vi "Write_Spreadsheet.vi"(0 "File_Path":path, 7 "Table":string[][](array[string]), 11 "Error_In":errorcluster) -> (15 "Error_Out":errorcluster)   [LabVIEW 2023, in "Custom_Sort_Library.lvlib"]
doc: "This VI Writes the given data to CSV file"
uses:
  Custom_Sort_Library.lvlib
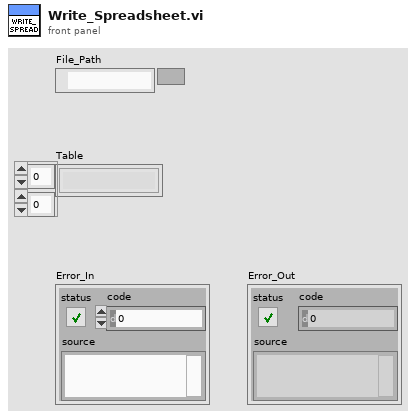
[diagram p1: front panel]
types:
  T1 = enum16{"open", "replace", "create", "open or create", "replace or create", "replace or create with confirmation"}
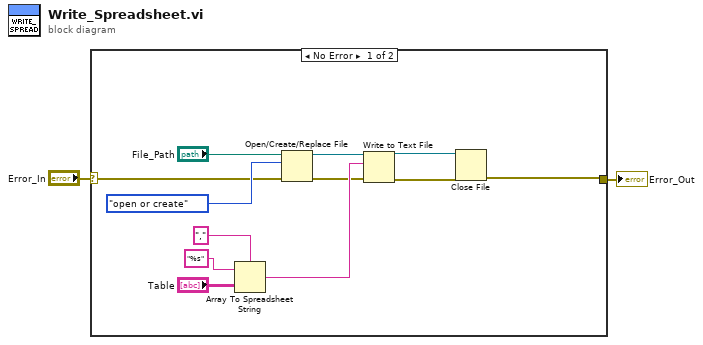
[diagram p0: block diagram]
diagram:
  n1 = case shown="No Error" "Error_In" {
    selector: "Error_In" -> [w9 w15]
    tunnel: [w4 w15] -> w2
    frame No Error {
      n2 = Array To Spreadsheet String(delimiter (Tab)=",", array="Table", 3:"%s" ("format string")) -> (spreadsheet string=w14:string)
      n3 = Open/Create/Replace File(file path (use dialog)="File_Path", error in=w9, operation (0:open)=T1."open or create") -> (refnum out=w13:refnum<file>, error out=w10:errorcluster)  [unwired: 3 in, 1 out]
      n4 = Write to Text File(file (use dialog)=w13, text=w14, error in=w10) -> (refnum out=w3:refnum<file>, error out=w5:errorcluster)  [unwired: 1 in, 1 out]
      n5 = Close File(refnum=w3, error in=w5) -> (error out=w4:errorcluster)  [unwired: 1 out]
    }
    frame Error {
    }
  }
  "Error_Out" <- w2
